vi "Build.vi"(0 "VIP In":refnum<class "VIP.lvclass">) -> (4 "VIP Out":refnum<class "VIP.lvclass">)   [LabVIEW 2017, in "CL_G3_VIComponentBuilder.lvlib" / "VIP.lvclass"]
doc: "Automates build with VI Package manager."
uses:
  VIP.lvclass
  C:/builds/Component BuilderBT/SrcDist/Exports/Exports/Export.lvclass
  Exports/Export.lvclass/Export.ctl
  Exports/Accessors/Read Export Build Specification.vi
  Exports/Accessors/Read Component Root path.vi
  Exports/Accessors/Write Exported Build Specification Path.vi
  Exports/Accessors/Read Exported Build Specification Path.vi
  Exports/Accessors/Read Component Export Dir.vi
  Exports/Accessors/Write Built Export's Full Path.vi
  Exports/Accessors/Write Export Operation Errors.vi
  Exports/Accessors/Read Export Operation Errors.vi
  <vilib>/Utility/file.llb/Is Path and Not Empty.vi
  <vilib>/Utility/libraryn.llb/Check if File or Folder Exists.vi
  Exports/Export.lvclass
  VIPM Utilities/CL_G3_VIPMUtilities.lvlib
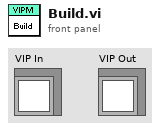
[diagram p1: front panel]
types:
  T1 = cluster{"Export":refnum<class "VIP.lvclass">, "Export's Source Folders":path[], "Library_Source_Folder":path, "Source Dummy Project Ref":refnum<vi>, "\"My Computer\" Project Ref ":refnum<vi>, "Temporary Export Location":path, "Export Definition File Path":path}
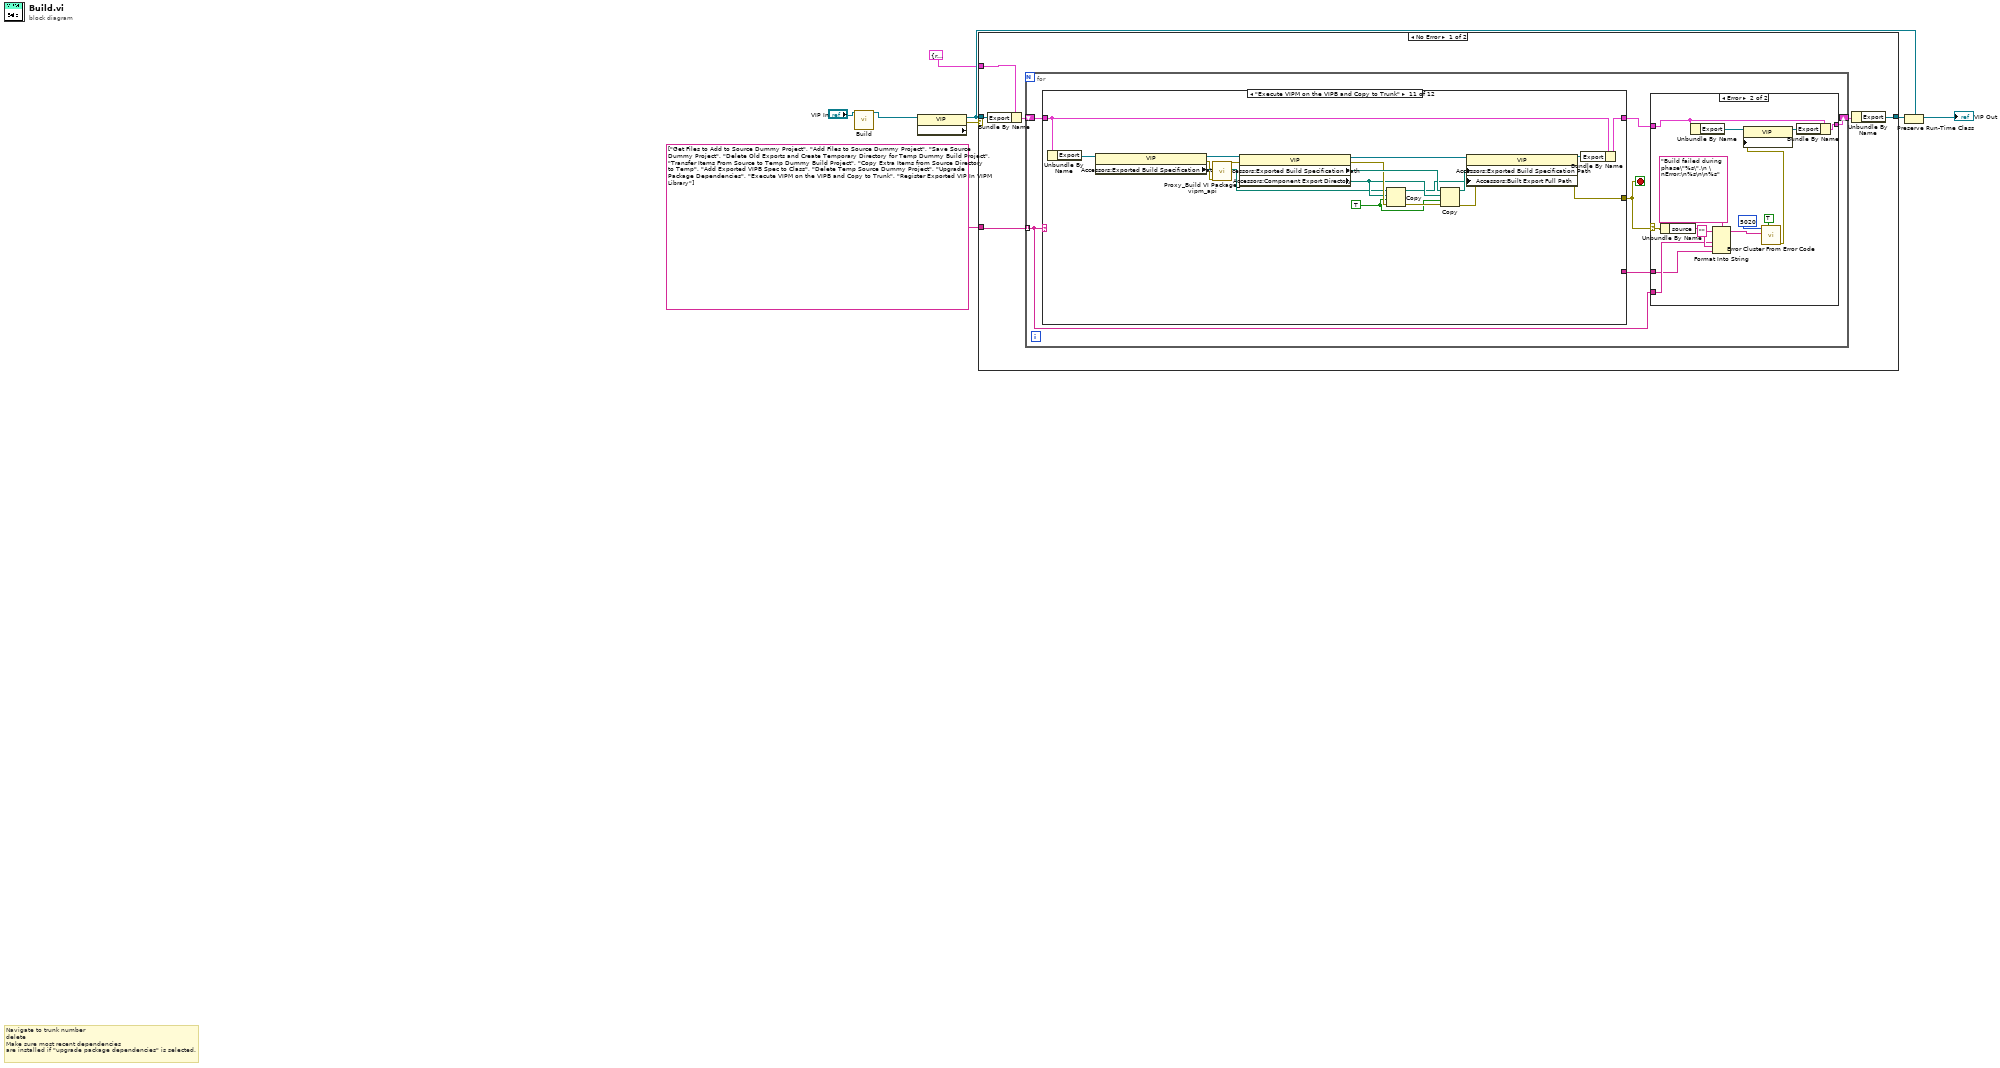
[diagram p0: block diagram]
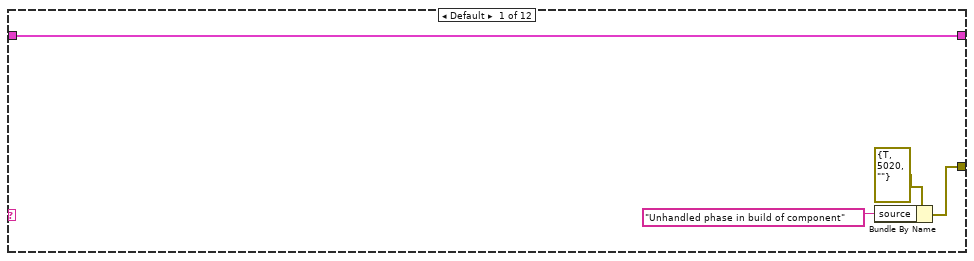
[diagram p3: hidden frame]
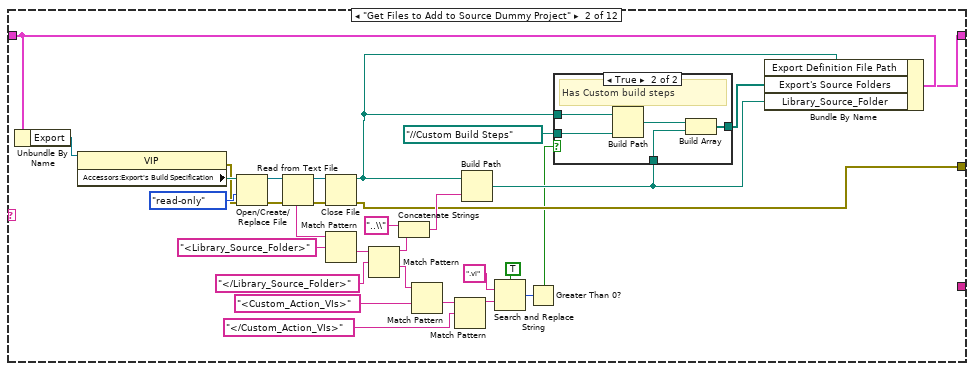
[diagram p4: hidden frame]
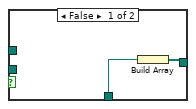
[diagram p5: hidden frame]
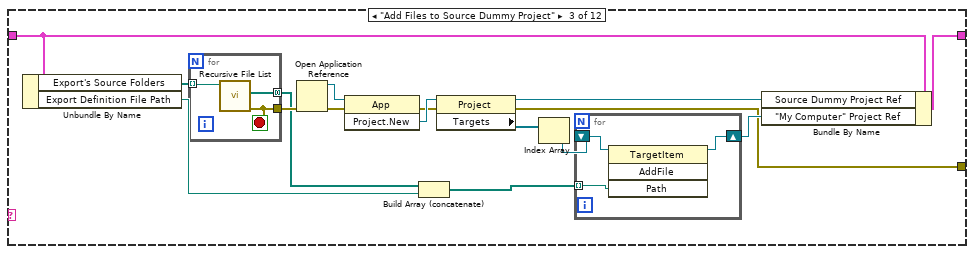
[diagram p6: hidden frame]
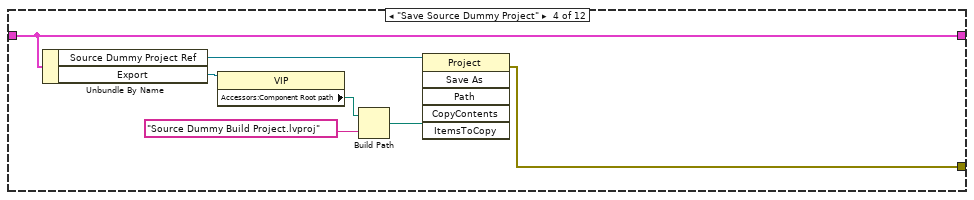
[diagram p7: hidden frame]
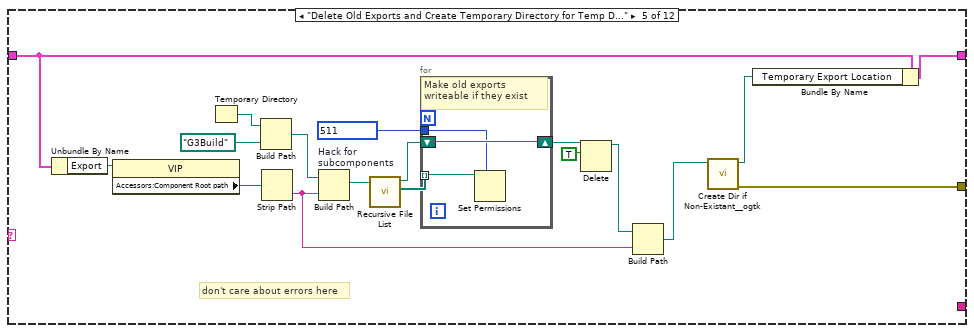
[diagram p8: hidden frame]
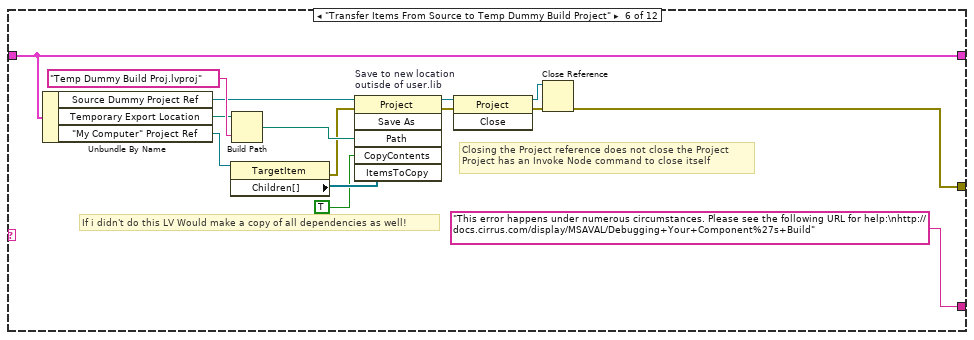
[diagram p9: hidden frame]
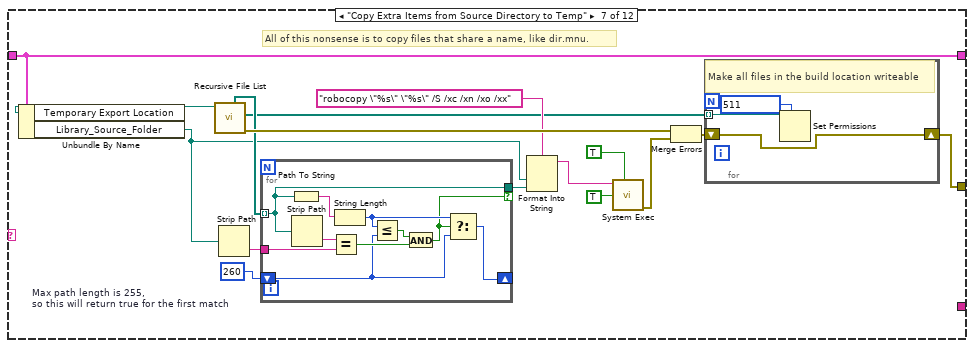
[diagram p10: hidden frame]
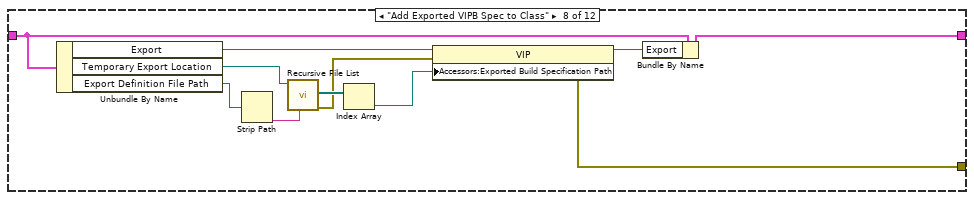
[diagram p11: hidden frame]
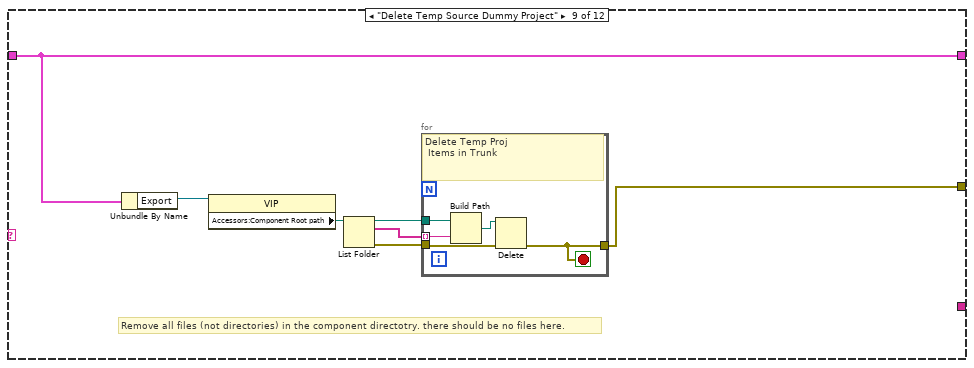
[diagram p12: hidden frame]
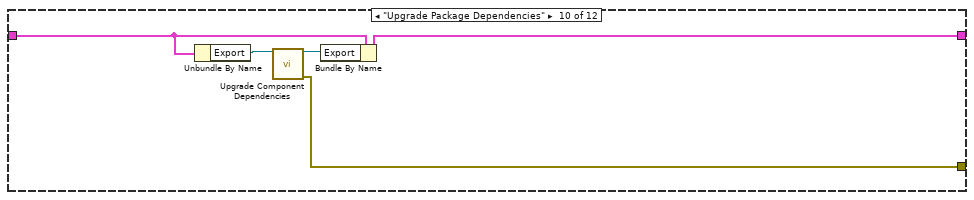
[diagram p13: hidden frame]
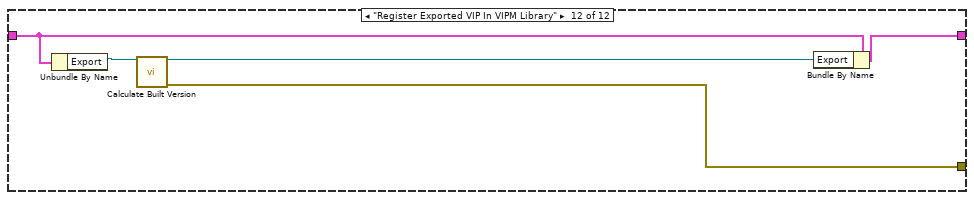
[diagram p14: hidden frame]
diagram:
  # "Navigate to trunk number \ndelete\nMake sure most recent dependencies\nare installed if \"upgrade package dependencies\" is selected."
  n1 = call-parent "Build.vi"("Export In"="VIP In") -> ("Export Out"=w1:refnum<class "VIP.lvclass">)  [unwired: 14 in]
  n2 = property class="VIP"(reference=w1) -> (reference out=w6:refnum<class "VIP.lvclass">, "Accessors:Merged Errors"=w5:errorcluster)  [unwired: 1 in, 1 out]
  n3 = case shown="No Error" w5 {
    tunnel: [w13 w224] -> w7
    tunnel: w6 -> [w11 w224]
    tunnel: string[] ["Get Files to Add to Source Dummy Project", "Add Files to Source Dummy Project", "Save Source Dummy Project", "Delete Old Exports and Create Temporary Directory for Temp Dummy Build Project", "Transfer Items From Source to Temp Dummy Build Project", "Copy Extra Items from Source Directory to Temp", "Add Exported VIPB Spec to Class", "Delete Temp Source Dummy Project", "Upgrade Package Dependencies", "Execute VIPM on the VIPB and Copy to Trunk", "Register Exported VIP In VIPM Library"] -> [w10 _]
    tunnel: T1 {"Export"=refnum, "Export's Source Folders"=[], "Library_Source_Folder"=path "", "Source Dummy Project Ref"=refnum, "\"My Computer\" Project Ref "=refnum, "Temporary Export Location"=path "", "Export Definition File Path"=path ""} -> [w9 _]
    frame No Error {
      n4 = Bundle By Name(cluster=w9, "Export"=w11) -> (w12:T1)
      n5 = for {
        tunnel: w10 -> [w16] mode=indexing
        shift-right: [w18] -> w14
        shift-left: w12 -> [w20]
        stop <- w17 stop-if-true
        n6 = case shown="\"Execute VIPM on the VIPB and Copy to Trunk\"" w16 {
          tunnel: w20 -> [w39 w70 w88 w105 w117 w142 w148 w181 w186 w199 w218 w223]
          tunnel: [w39 w55 w85 w105 w114 w142 w148 w180 w186 w198 w214 w222] -> w19
          tunnel: [w36 w56 w80 w103 w109 w133 w143 w174 w185 w195 w203 w220] -> w17
          tunnel: [_ _ _ _ _ "This error happens under numerous circumstances. Please see the following URL for help:\nhttp://docs.cirrus.com/display/MSAVAL/Debugging+Your+Component%27s+Build" ("format string") _ _ _ _ _ _] -> w15
          frame Default {
            n7 = Bundle By Name(cluster=errorcluster {"status"=TRUE, "code"=5020, "source"=""} ("error out"), "source"="Unhandled phase in build of component" ("format string")) -> (w36:errorcluster)
          }
          frame "Get Files to Add to Source Dummy Project" {
            n8 = Unbundle By Name(w70) -> ("Export"=w69:refnum<class "VIP.lvclass">)
            n9 = property class="VIP"(reference=w69) -> (error out=w51:errorcluster, "Accessors:Export's Build Specification"=w52:path)  [unwired: 1 in, 1 out]
            n10 = Open/Create/Replace File(file path (use dialog)=w52, error in=w51, access (0:read/write)=enum16{"read/write", "read-only", "write-only"}."read-only") -> (refnum out=w68:refnum<file>, error out=w61:errorcluster)  [unwired: 3 in, 1 out]
            n11 = Read from Text File(file (use dialog)=w68, error in=w61) -> (refnum out=w62:refnum<file>, text=w67:string, error out=w60:errorcluster)  [unwired: 2 in, 1 out]
            n12 = Close File(refnum=w62, error in=w60) -> (path=w50:path, error out=w56:errorcluster)
            n13 = Match Pattern(string=w67, regular expression="<Library_Source_Folder>") -> (after substring=w65:string)  [unwired: 1 in, 3 out]
            n14 = Match Pattern(string=w65, regular expression="</Library_Source_Folder>") -> (before substring=w59:string, after substring=w43:string)  [unwired: 1 in, 2 out]
            n15 = Concatenate Strings("..\\" ("string"), w59) -> (w58:string)
            n16 = Match Pattern(string=w43, regular expression="<Custom_Action_VIs>") -> (after substring=w48:string)  [unwired: 1 in, 3 out]
            n17 = Match Pattern(string=w48, regular expression="</Custom_Action_VIs>") -> (before substring=w46:string)  [unwired: 1 in, 3 out]
            n18 = Build Path(base path=w50, name or relative path=w58) -> (appended path=w53:path)
            n19 = Search and Replace String(case sensitive?=TRUE ("ignore case? (F)"), input string=w46, search string=".vi") -> (number of replacements=w42:i32)  [unwired: 5 in, 3 out]
            n20 = Greater Than 0?(x=w42) -> (x > 0?=w41:bool)
            n21 = case shown="True" w41 {
              tunnel: [w71 w77] -> w54
              tunnel: w53 -> [w72 w76]
              tunnel: w50 -> [_ w74]
              tunnel: path "../../Custom Build Steps" ("path") -> [_ w73]
              frame False {
                n22 = Build Array(w72) -> (w71:path[])
              }
              frame True {
                # "Has Custom build steps"
                n23 = Build Path(base path=w74, name or relative path=w73) -> (appended path=w75:path)
                n24 = Build Array(w75, w76) -> (w77:path[])
              }
            }
            n25 = Bundle By Name(cluster=w70, "Export Definition File Path"=w50, "Export's Source Folders"=w54, "Library_Source_Folder"=w53) -> (w55:T1)
          }
          frame "Add Files to Source Dummy Project" {
            n26 = Unbundle By Name(w88) -> ("Export's Source Folders"=w87:path[], "Export Definition File Path"=w78:path)
            n27 = for {
              tunnel: [w99] -> w81 mode=concatenating
              tunnel: w87 -> [w98] mode=indexing
              tunnel: [w97] -> w86
              stop <- w97 stop-if-true
              n28 = call <vilib>:"Recursive File List.vi"("Folder Path"=w98) -> ("error out"=w97:errorcluster, "All Files in Dir"=w99:path[])  [unwired: 6 in, 3 out]
            }
            n29 = Open Application Reference(8:w86) -> (0:w91:errorcluster, 3:w93:refnum<vi>)  [unwired: 3 in]
            n30 = invoke class="App" method="Project.New"(reference=w93, error in=w91) -> (error out=w89:errorcluster, "Project:New"=w90:refnum<vi>)  [unwired: 1 in, 1 out]
            n31 = Build Array (concatenate)(w81, w78) -> (w79:path[])
            n32 = property class="Project"(reference=w90, error in=w89) -> (reference out=w83:refnum<vi>, error out=w80:errorcluster, "Targets"=w92:refnum<vi>[])
            n33 = Index Array(array=w92) -> (element=w84:refnum<vi>)  [unwired: 1 in]
            n34 = for {
              tunnel: w79 -> [w94] mode=indexing
              shift-right: [w95] -> w82
              shift-left: w84 -> [w96]
              n35 = invoke class="TargetItem" method="AddFile"(reference=w96, "Path"=w94) -> (reference out=w95:refnum<vi>)  [unwired: 2 in, 3 out]
            }
            n36 = Bundle By Name(cluster=w88, "Source Dummy Project Ref"=w83, "\"My Computer\" Project Ref"=w82) -> (w85:T1)
          }
          frame "Save Source Dummy Project" {
            n37 = Unbundle By Name(w105) -> ("Source Dummy Project Ref"=w102:refnum<vi>, "Export"=w101:refnum<class "VIP.lvclass">)
            n38 = property class="VIP"(reference=w101) -> ("Accessors:Component Root path"=w100:path)  [unwired: 1 in, 2 out]
            n39 = Build Path(base path=w100, name or relative path="Source Dummy Build Project.lvproj" ("pattern")) -> (appended path=w106:path)
            n40 = invoke class="Project" method="Save As"(reference=w102, "Path"=w106) -> (error out=w103:errorcluster)  [unwired: 4 in, 5 out]
          }
          frame "Delete Old Exports and Create Temporary Directory for Temp Dummy Build Project" {
            # "don't care about errors here"
            n41 = Unbundle By Name(w117) -> ("Export"=w108:refnum<class "VIP.lvclass">)
            n42 = property class="VIP"(reference=w108) -> ("Accessors:Component Root path"=w107:path)  [unwired: 1 in, 2 out]
            n43 = Temporary Directory() -> (w123:path)
            n44 = Build Path(base path=w123, name or relative path=path "G3Build" ("path")) -> (appended path=w122:path)
            n45 = Strip Path(path=w107) -> (name=w113:string)  [unwired: 1 out]
            n46 = Build Path "Hack for \nsubcomponents"(base path=w122, name or relative path=w113) -> (appended path=w120:path)
            n47 = call <vilib>:"Recursive File List.vi"("Folder Path"=w120) -> ("All Files in Dir"=w121:path[], "dup Folder Path"=w119:path)  [unwired: 6 in, 3 out]
            n48 = for {
              tunnel: w121 -> [w127] mode=indexing
              shift-right: [w126] -> w116
              shift-left: w119 -> [w126]
              tunnel: i16 511 ("permissions") -> [w125]
              # "Make old exports writeable if they exist"
              n49 = Set Permissions(7:w125, 11:w127) -> ()  [unwired: 3 in, 2 out]
            }
            n50 = Delete(path (use dialog)=w116, entire hierarchy (F)=TRUE) -> (deleted path=w112:path)  [unwired: 3 in, 2 out]
            n51 = Build Path(base path=w112, name or relative path=w113) -> (appended path=w111:path)
            n52 = call <userlib>:"Create Dir if Non-Existant__ogtk.vi"("Directory Path"=w111) -> ("error out"=w109:errorcluster, "dup Directory Path"=w110:path)  [unwired: 8 in, 1 out]
            n53 = Bundle By Name(cluster=w117, "Temporary Export Location"=w110) -> (w114:T1)
          }
          frame "Transfer Items From Source to Temp Dummy Build Project" {
            # "Closing the Project reference does not close the Project\nProject has an Invoke Node command to close itself"
            # "If i didn't do this LV Would make a copy of all dependencies as well!"
            n54 = Unbundle By Name(w142) -> ("Source Dummy Project Ref"=w137:refnum<vi>, "Temporary Export Location"=w136:path, "\"My Computer\" Project Ref"=w139:refnum<vi>)
            n55 = property class="TargetItem"(reference=w139) -> (error out=w135:errorcluster, "Children[]"=w138:refnum<vi>[])  [unwired: 1 in, 1 out]
            n56 = Build Path(base path=w136, name or relative path="Temp Dummy Build Proj.lvproj") -> (appended path=w140:path)
            n57 = invoke on="Save to new location \noutisde of user.lib" class="Project" method="Save As"(reference=w137, error in=w135, "Path"=w140, "CopyContents"=TRUE ("Copy contents?"), "ItemsToCopy"=w138) -> (reference out=w129:refnum<vi>, error out=w134:errorcluster)  [unwired: 1 in, 4 out]
            n58 = invoke class="Project" method="Close"(reference=w129, error in=w134) -> (reference out=w128:refnum<vi>, error out=w130:errorcluster)  [unwired: 1 in, 1 out]
            n59 = Close Reference(reference=w128, error in (no error)=w130) -> (error out=w133:errorcluster)
          }
          frame "Copy Extra Items from Source Directory to Temp" {
            w149 = 260  # Max path length is 255,  so this will return true for the first match
            # "All of this nonsense is to copy files that share a name, like dir.mnu."
            n60 = Unbundle By Name(w148) -> ("Temporary Export Location"=w147:path, "Library_Source_Folder"=w144:path)
            n61 = call <vilib>:"Recursive File List.vi"("Folder Path"=w147) -> ("error out"=w158:errorcluster, "All Files in Dir"=w146:path[], "All Folders"=w152:path[])  [unwired: 6 in, 2 out]
            n62 = Strip Path(path=w144) -> (name=w151:string)  [unwired: 1 out]
            n63 = for {
              tunnel: w152 -> [w163] mode=indexing
              tunnel: w151 -> [w170]
              shift-right: [w164] -> _
              shift-left: w149 -> [w165]
              tunnel: [w163] -> w150 if=w162
              n64 = Path To String(path=w163) -> (string=w169:string)
              n65 = Strip Path(path=w163) -> (name=w171:string)  [unwired: 1 out]
              n66 = Equal?(x=w171, y=w170) -> (x = y?=w167:bool)
              n67 = String Length(string=w169) -> (length=w166:i32)
              n68 = Less Or Equal?(x=w166, y=w165) -> (x <= y?=w168:bool)
              n69 = And(x=w168, y=w167) -> (x .and. y?=w162:bool)
              n70 = Select(t=w166, s=w162, f=w165) -> (s? t:f=w164:i32)
            }
            n71 = Format Into String(format string="robocopy \"%s\" \"%s\" /S /xc /xn /xo /xx" ("command line"), w144, w150) -> (resulting string=w156:string)  [unwired: 2 in, 1 out]
            n72 = call <vilib>:"System Exec.vi"("run minimized? (F)"=TRUE, "wait until completion? (T)"=TRUE, "command line"=w156) -> ("error out"=w154:errorcluster)  [unwired: 5 in, 3 out]
            n73 = Merge Errors(w158, w154) -> (w145:errorcluster)
            n74 = for {
              tunnel: w146 -> [w160] mode=indexing
              shift-right: [w159] -> w143
              shift-left: w145 -> [w159]
              # "Make all files in the build location writeable"
              n75 = Set Permissions(7:i16 511 ("permissions"), 11:w160) -> ()  [unwired: 3 in, 2 out]
            }
          }
          frame "Add Exported VIPB Spec to Class" {
            n76 = Unbundle By Name(w181) -> ("Export"=w173:refnum<class "VIP.lvclass">, "Temporary Export Location"=w177:path, "Export Definition File Path"=w172:path)
            n77 = Strip Path(path=w172) -> (name=w176:string)  [unwired: 1 out]
            n78 = call <vilib>:"Recursive File List.vi"("pattern"=w176, "Folder Path"=w177) -> ("error out"=w175:errorcluster, "All Files in Dir"=w182:path[])  [unwired: 5 in, 3 out]
            n79 = Index Array(array=w182) -> (element=w178:path)  [unwired: 1 in]
            n80 = property class="VIP"(reference=w173, error in=w175, "Accessors:Exported Build Specification Path"=w178) -> (reference out=w179:refnum<class "VIP.lvclass">, error out=w174:errorcluster)
            n81 = Bundle By Name(cluster=w181, "Export"=w179) -> (w180:T1)
          }
          frame "Delete Temp Source Dummy Project" {
            # "Remove all files (not directories) in the component directotry. there should be no files here."
            n82 = Unbundle By Name(w186) -> ("Export"=w184:refnum<class "VIP.lvclass">)
            n83 = property class="VIP"(reference=w184) -> ("Accessors:Component Root path"=w183:path)  [unwired: 1 in, 2 out]
            n84 = List Folder(path=w183) -> (path out=w187:path, filenames=w189:string[], error out=w188:errorcluster)  [unwired: 3 in, 1 out]
            n85 = for {
              tunnel: w189 -> [w194] mode=indexing
              tunnel: w187 -> [w193]
              tunnel: w188 -> [w191]
              tunnel: [w190] -> w185
              stop <- w190 stop-if-true
              # "Delete Temp Proj\n Items in Trunk"
              n86 = Build Path(base path=w193, name or relative path=w194) -> (appended path=w192:path)
              n87 = Delete(path (use dialog)=w192, error in=w191) -> (error out=w190:errorcluster)  [unwired: 3 in, 2 out]
            }
          }
          frame "Upgrade Package Dependencies" {
            n88 = Unbundle By Name(w199) -> ("Export"=w197:refnum<class "VIP.lvclass">)
            n89 = call-dynamic "Upgrade Component Dependencies.vi"("VIPM In"=w197) -> ("VIPM Out"=w196:refnum<class "VIP.lvclass">, "error out"=w195:errorcluster)  [unwired: 13 in]
            n90 = Bundle By Name(cluster=w199, "Export"=w196) -> (w198:T1)
          }
          frame "Execute VIPM on the VIPB and Copy to Trunk" {
            w210 = TRUE ("overwrite (F)")
            n91 = Unbundle By Name(w218) -> ("Export"=w217:refnum<class "VIP.lvclass">)
            n92 = property class="VIP"(reference=w217) -> (reference out=w201:refnum<class "VIP.lvclass">, error out=w215:errorcluster, "Accessors:Exported Build Specification Path"=w216:path)  [unwired: 1 in]
            n93 = call "Proxy_Build VI Package_vipm_api.vi"("error in (no error)"=w215, "Path to VIPB File"=w216) -> ("error out"=w204:errorcluster, "Build Output"=w205:path)  [unwired: 8 in]
            n94 = property class="VIP"(reference=w201, error in=w204) -> (reference out=w209:refnum<class "VIP.lvclass">, error out=w211:errorcluster, "Accessors:Exported Build Specification Path"=w212:path, "Accessors:Component Export Directory"=w206:path)
            n95 = Copy(8:w211, 9:w210, 10:w206, 11:w205) -> (0:w213:errorcluster, 3:w200:path)  [unwired: 1 in, 1 out]
            n96 = Copy(8:w213, 9:w210, 10:w206, 11:w212) -> (0:w207:errorcluster, 3:w208:path)  [unwired: 1 in, 1 out]
            n97 = property class="VIP"(reference=w209, error in=w207, "Accessors:Exported Build Specification Path"=w208, "Accessors:Built Export Full Path"=w200) -> (reference out=w202:refnum<class "VIP.lvclass">, error out=w203:errorcluster)
            n98 = Bundle By Name(cluster=w218, "Export"=w202) -> (w214:T1)
          }
          frame "Register Exported VIP In VIPM Library" {
            n99 = Unbundle By Name(w223) -> ("Export"=w219:refnum<class "VIP.lvclass">)
            n100 = call-dynamic "Calculate Built Version.vi"("VIP in"=w219) -> ("VIP out"=w221:refnum<class "VIP.lvclass">, "error out"=w220:errorcluster)  [unwired: 13 in]
            n101 = Bundle By Name(cluster=w223, "Export"=w221) -> (w222:T1)
          }
        }
        n102 = case shown="Error" w17 {
          selector: w17 -> [_ w27]
          tunnel: w19 -> [w21 w25]
          tunnel: [w21 w35] -> w18
          tunnel: w16 -> [_ w28]
          tunnel: w15 -> [_ w26]
          frame No Error {
          }
          frame Error {
            n103 = Unbundle By Name(w27) -> ("source"=w29:string)
            n104 = Unbundle By Name(w25) -> ("Export"=w24:refnum<class "VIP.lvclass">)
            n105 = Format Into String(format string="Build failed during phase\"%s\".\n \nError:\n%s\n\n%s" ("error message (\"\")"), initial string="", w28, w29, w26) -> (resulting string=w32:string)  [unwired: 1 in, 1 out]
            n106 = call <vilib>:"Error Cluster From Error Code.vi"("show call chain? (False)"=TRUE, "error message (\"\")"=w32, "error code (0)"=5020) -> ("error out"=w22:errorcluster)  [unwired: 6 in]
            n107 = property class="VIP"(reference=w24, "Accessors:Merged Errors"=w22) -> (reference out=w23:refnum<class "VIP.lvclass">)  [unwired: 1 in, 1 out]
            n108 = Bundle By Name(cluster=w25, "Export"=w23) -> (w35:T1)
          }
        }
      }
      n109 = Unbundle By Name(w14) -> ("Export"=w13:refnum<class "VIP.lvclass">)
    }
    frame Error {
    }
  }
  n110 = Preserve Run-Time Class(object in=w7, 2:w6) -> (object out=→"VIP Out":refnum<class "VIP.lvclass">)  [unwired: 1 in, 1 out]
